vi "convert_to_DD.vi"(11 "Array":waveform(dbl)[][](array[waveform])) -> (3 "Dynamic Data":dynamicdata(waveform))   [LabVIEW 2019]
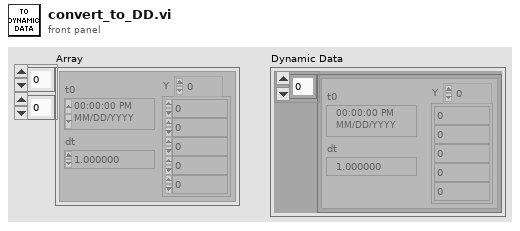
[diagram p1: front panel]
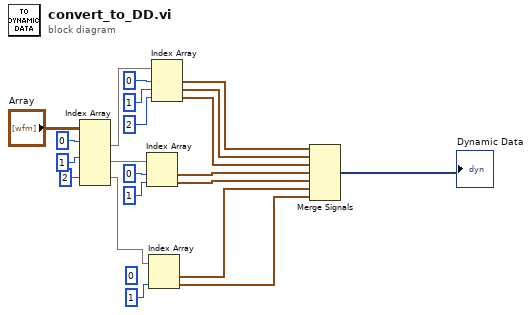
[diagram p0: block diagram]
diagram:
  (unwired) 0 ("index")
  n1 = Index Array(array="Array", index (row) #1=0 ("index (row)"), index (row) #2=1 ("index (row)"), index (row) #3=2 ("index (row)")) -> (element #1=w6:waveform(dbl)[], element #2=w7:waveform(dbl)[], element #3=w3:waveform(dbl)[])  [unwired: 3 in]
  n2 = Index Array(array=w7, index #1=0 ("index"), index #2=1 ("index")) -> (element #1=w8:waveform(dbl), element #2=w18:waveform(dbl))
  n3 = Index Array(array=w3, index #2=1 ("index")) -> (element #1=w2:waveform(dbl), element #2=w1:waveform(dbl))  [unwired: 1 in]
  n4 = Index Array(array=w6, index #1=0 ("index"), index #2=1 ("index"), index #3=2 ("index")) -> (element #1=w19:waveform(dbl), element #2=w9:waveform(dbl), element #3=w15:waveform(dbl))
  n5 = Merge Signals(w19, w9, w15, w8, w18, w2, w1) -> (→"Dynamic Data":dynamicdata)
